vi "Flatten Value.vi"(8 "Error In":errorcluster, 11 "Path In":refnum<class "Path.lvclass">) -> (0 "Error Out":errorcluster, 1 "Value":string, 3 "Path Out":refnum<class "Path.lvclass">)   [LabVIEW 2020, in "NI_VIAnCFGDataStructure.lvlib" / "Path.lvclass"]
uses:
  <vilib>/addons/analyzer/VIAnCFGDataStructure/Data Types/Path/Path.lvclass
  <vilib>/addons/analyzer/VIAnCFGDataStructure/Data Types/Path/Path.lvclass/Path.ctl
  <vilib>/addons/analyzer/VIAnCFGDataStructure/Tree Manager/API/Generate Hash.vi
  <vilib>/addons/analyzer/VIAnCFGDataStructure/Tree Manager/Tree.lvclass
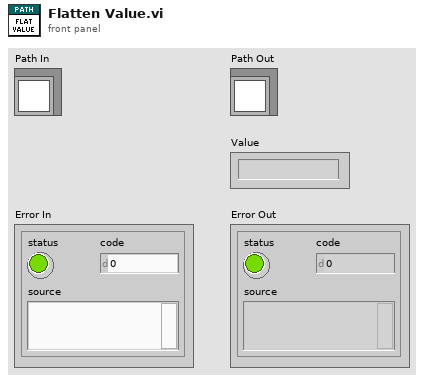
[diagram p1: front panel]
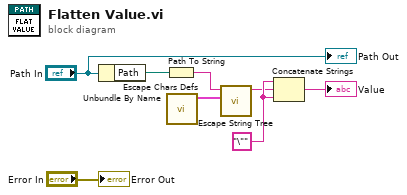
[diagram p0: block diagram]
diagram:
  w5 = "\"" ("string")
  n1 = Unbundle By Name("Path In") -> ("Path"=w8:path)
  n2 = Path To String(path=w8) -> (string=w3:string)
  n3 = call <vilib>:"Escape Chars Defs.vi"() -> ("Escapes"=w2:cluster{"String":string, "Escape":string}[])  [unwired: 11 in]
  n4 = call <vilib>:"Escape String Tree.vi"("Escapes"=w2, "String In"=w3) -> ("String Out"=w1:string)  [unwired: 9 in]
  n5 = Concatenate Strings(w5, w1, w5) -> (→"Value":string)
  "Path Out" <- "Path In"
  "Error Out" <- "Error In"
